vi "Compile with Pair Array.vi"(6 "Loader":refnum<class "Loader.lvclass">, 7 "Data":refnum<class "Pair.lvclass">[](array[class]), 8 "Error In":errorcluster, 10 "Hooks In":T1, 11 "Input":string) -> (0 "Error Out":errorcluster, 2 "Hooks Out":T1, 3 "Output":string)   [LabVIEW 2018, in "Toolkit.lvlib"]
doc: "Compiles a Mustache template using the supplied data and their types to control the rendering process. The type fo data for each tag and key determines the rendering behavior of the node in the syntax tree, so LabVIEW classes are provided to convert LabVIEW values and represent the different data types.\n\n<b>Input</b> - A logic-free Mustache template as a string that will be compiled, or rendered, to the output based on the data provided.\n\n<B>Data</B> - Mustache data represented either as an array of key-value pairs, an array of key-value string clusters, or a generic Datum object. The rendering of a Mustache template is dependent on the existence and type of data provided at compilation.\n\n<B>Loader</B> - Responsible for importing, or including, other Mustache templates within the root template.\n\n<B>Output</B> - A string representing the completely lexed, parsed, and rendered Mustache template based on the supplied data's types and values."
uses:
  Toolkit.lvlib
  Low-Level/Loaders/Loader/Loader.lvclass
  Data/Pair/Pair.lvclass
  Low-Level/Type Definitions/Hooks.ctl
  Hooks/Render/Delimiter/Delimiter.lvclass
  Hooks/Render/Process/Process.lvclass
  Hooks/Render/Section/Section.lvclass
  Hooks/Render/Variable/Variable.lvclass
  Hooks/Render/Comment/Comment.lvclass
  Hooks/Render/Node/Node.lvclass
  Hooks/Render/Partial/Partial.lvclass
  Hooks/Render/Text/Text.lvclass
  Hooks/Compile/Process/Process.lvclass
  Data/Map/Map.lvclass
  D:/Users/cfield/Code/Field R&D Services/Labstache/src/Toolkit/Data/Datum/Datum.lvclass
  Data/Map/Support/From Pair Array.vi
  Low-Level/Support/Lex String.vi
  Low-Level/Support/Render to String.vi
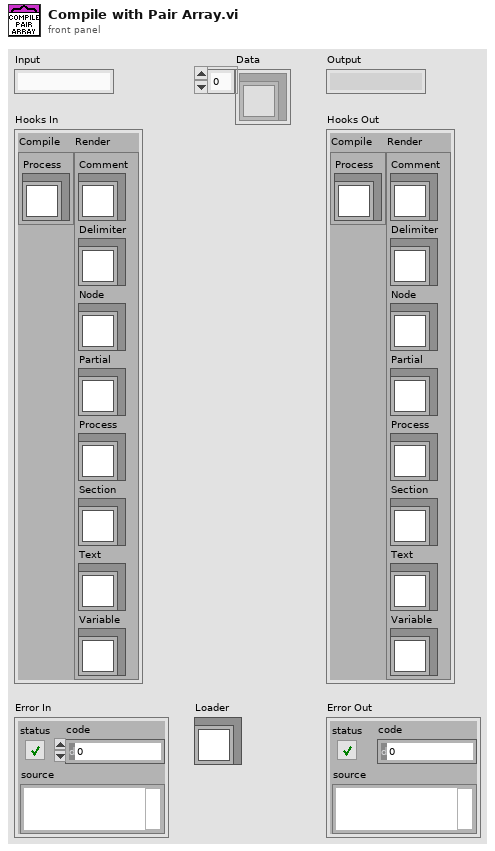
[diagram p1: front panel]
types:
  T1 = typedef "Toolkit.lvlib/Hooks.ctl" = cluster{"Compile":cluster{"Process":refnum<class "Process.lvclass">}, "Render":cluster{"Comment":refnum<class "Comment.lvclass">, "Delimiter":refnum<class "Delimiter.lvclass">, "Node":refnum<class "Node.lvclass">, "Partial":refnum<class "Partial.lvclass">, "Process":refnum<class "Process.lvclass">, "Section":refnum<class "Section.lvclass">, "Text":refnum<class "Text.lvclass">, "Variable":refnum<class "Variable.lvclass">}}
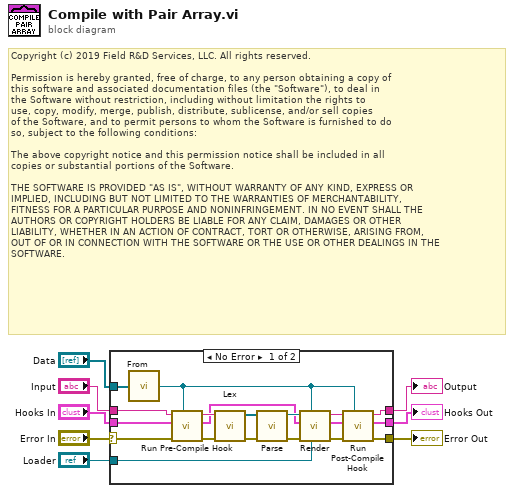
[diagram p0: block diagram]
diagram:
  # "Copyright (c) 2019 Field R&D Services, LLC. All rights reserved.\n\nPermission is hereby granted, free of charge, to any person obtaining a copy of\nthis software and associated documentation files (the \"Software\"), to deal in\nthe Software without restriction, including without limitation the rights to\nuse, copy, modify, merge, publish, distribute, sublicense, and/or sell copies\nof the Software, and to permit persons to whom the Software is furnished to do\nso, subject to the following conditions:\n\nThe above copyright notice and this permission notice shall be included in all\ncopies or substantial portions of the Software.\n\nTHE SOFTWARE IS PROVIDED \"AS IS\", WITHOUT WARRANTY OF ANY KIND, EXPRESS OR\nIMPLIED, INCLUDING BUT NOT LIMITED TO THE WARRANTIES OF MERCHANTABILITY,\nFITNESS FOR A PARTICULAR PURPOSE AND NONINFRINGEMENT. IN NO EVENT SHALL THE\nAUTHORS OR COPYRIGHT HOLDERS BE LIABLE FOR ANY CLAIM, DAMAGES OR OTHER\nLIABILITY, WHETHER IN AN ACTION OF CONTRACT, TORT OR OTHERWISE, ARISING FROM,\nOUT OF OR IN CONNECTION WITH THE SOFTWARE OR THE USE OR OTHER DEALINGS IN THE\nSOFTWARE."
  n1 = case shown="No Error" "Error In" {
    selector: "Error In" -> [w18 w29]
    tunnel: [w10 w29] -> w8
    tunnel: "Input" -> [w21 w30]
    tunnel: [w13 w30] -> w6
    tunnel: "Loader" -> [w22 _]
    tunnel: "Data" -> [w23 _]
    tunnel: "Hooks In" -> [w17 w28]
    tunnel: [w9 w28] -> w1
    frame No Error {
      n2 = call-poly "From.vi"("Pairs"=w23) -> ("Map"=w12:refnum<class "Map.lvclass">)  [unwired: 1 in]
      n3 = call "Run Pre-Compile Hook.vi"("Datum"=w12, "Error In"=w18, "Hooks In"=w17, "Input In"=w21) -> ("Error Out"=w19:errorcluster, "Hooks Out"=w16:T1, "Input Out"=w20:string)  [unwired: 5 in]
      n4 = call-poly "Lex.vi"("Error In"=w19, "Input"=w20) -> ("Error Out"=w24:errorcluster, "Tokens"=w27:refnum<class "Token.lvclass">[])  [unwired: 8 in]
      n5 = call "Parse.vi"("Error In"=w24, "Tokens"=w27) -> ("Error Out"=w25:errorcluster, "Abstract Syntax Tree"=w26:refnum<class "Root.lvclass">)  [unwired: 8 in]
      n6 = call-poly "Render.vi"("Loader"=w22, "Data"=w12, "Error In"=w25, "Hooks In"=w16, "Abstract Syntax Tree"=w26) -> ("Error Out"=w11:errorcluster, "Hooks Out"=w15:T1, "Output"=w14:string)  [unwired: 4 in]
      n7 = call "Run Post-Compile Hook.vi"("Datum"=w12, "Error In"=w11, "Hooks In"=w15, "Output In"=w14) -> ("Error Out"=w10:errorcluster, "Hooks Out"=w9:T1, "Output Out"=w13:string)  [unwired: 5 in]
    }
    frame Error {
    }
  }
  "Error Out" <- w8
  "Output" <- w6
  "Hooks Out" <- w1
